vi "noindexString.vi"() -> ()   [LabVIEW 2020]
panel:
  out "number":u64[](array[numeric]) format="%.0x"
  out "Array":string[](array[string])
  in  "String":string
  out "Batch Length":i32
  out "Actual Bitrate kHz 2":i32=1000
  out "dup Cheetah Handle":i32
  out "Total Shifted Out":i32
  out "Actual Bitrate kHz":i32=1000
  out "error out":errorcluster
  in  "Rds per Sec":dbl=2000.0 max=2000000000.0
  out "SDO":u64[](array[numeric]) format="%x"
  in  "SCLK (kHz)":i32=2000 min=0
  out "Cheetah Handle":i32
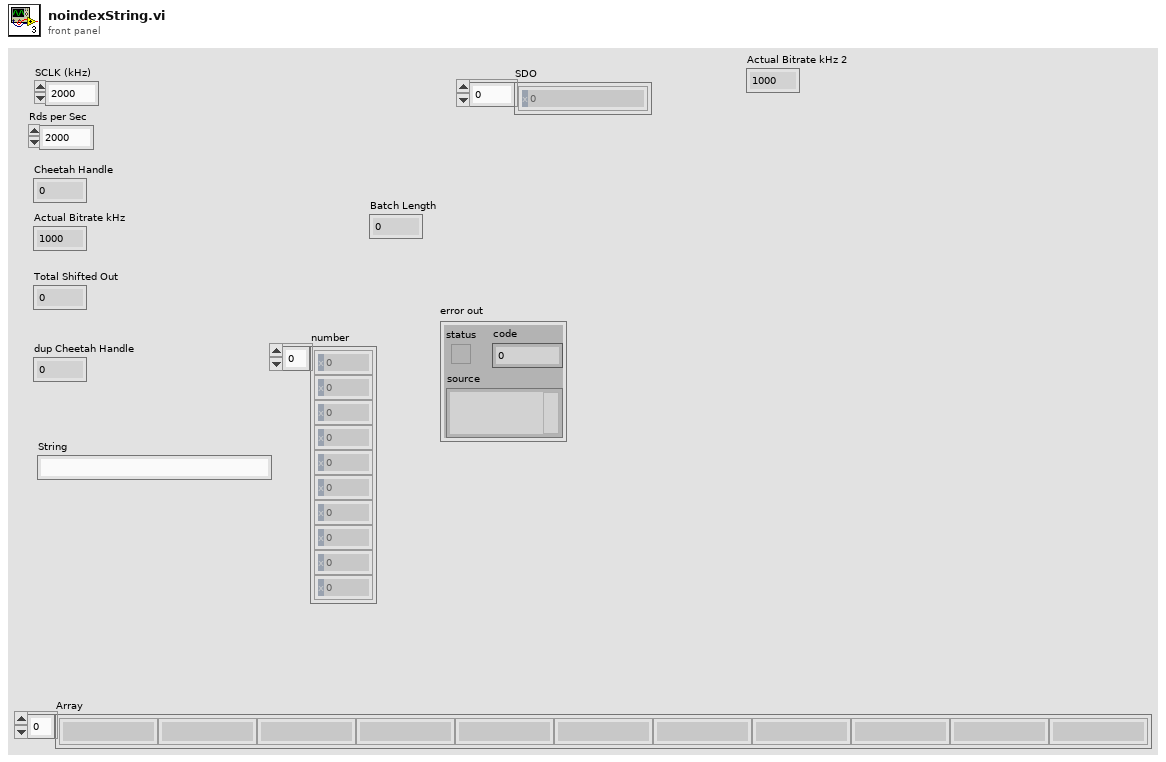
[diagram p1: front panel]
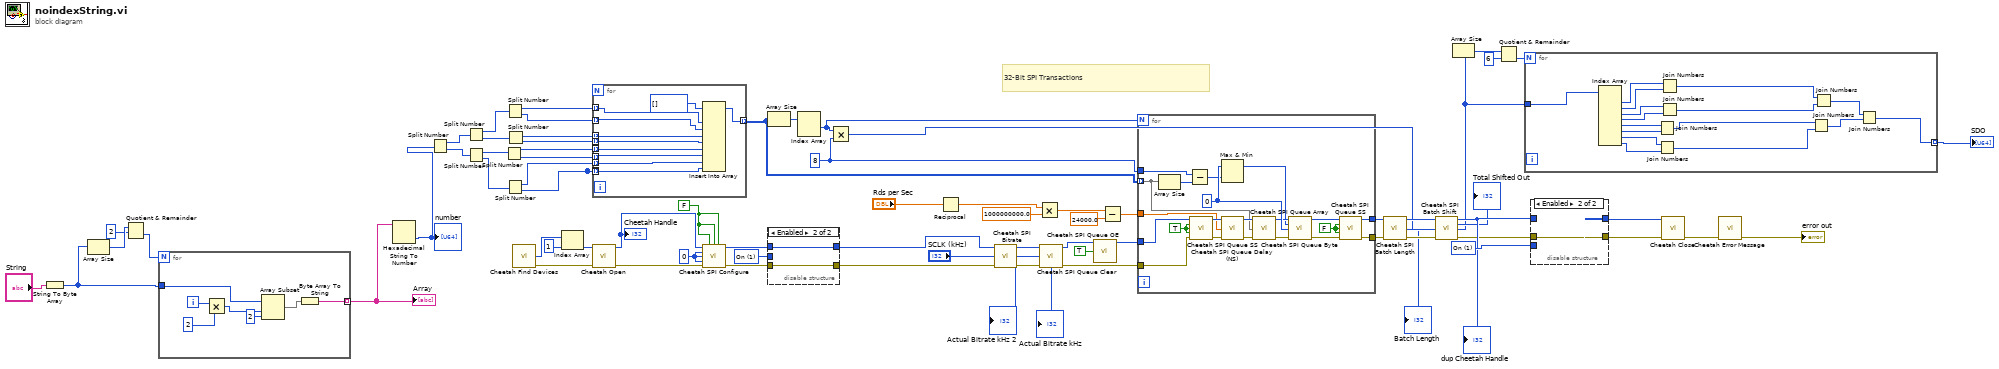
[diagram p0: block diagram]
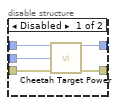
[diagram p2: hidden frame]
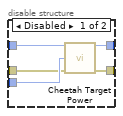
[diagram p3: hidden frame]
diagram:
  w26 = 8 ("y")
  w51 = u16 1 items=["Off", "On", "Query"] ("Requested Configuration (2: Query)")
  w52 = u16 1 items=["Off", "On", "Query"] ("Requested Configuration (2: Query)")
  w67 = FALSE
  w69 = 0
  # "32-Bit SPI Transactions"
  n1 = String To Byte Array(string="String") -> (unsigned byte array=w6:u8[])
  n2 = Array Size(array=w6) -> (size(s)=w5:i32)
  n3 = Quotient & Remainder(x=w5, y=2) -> (floor(x/y)=w3:i32)  [unwired: 1 out]
  n4 = for {
    N: w3 -> [_]
    tunnel: w6 -> [w78]
    tunnel: [w73] -> w2 mode=indexing
    i -> [w77]
    n5 = Multiply(x=w77, y=2) -> (x*y=w75:i32)
    n6 = Array Subset(array=w78, index=w75, length=2) -> (w72:u8[])
    n7 = Byte Array To String(unsigned byte array=w72) -> (string=w73:string)
  }
  "Array" <- w2
  n8 = Hexadecimal String To Number(string=w2) -> (number=w1:u32[])  [unwired: 2 in, 1 out]
  "number" <- w1
  n9 = Split Number(x=w1) -> (hi(x)=w37:u16[], lo(x)=w36:u16[])
  n10 = Split Number(x=w37) -> (hi(x)=w14:u8[], lo(x)=w13:u8[])
  n11 = Split Number(x=w36) -> (hi(x)=w16:u8[], lo(x)=w15:u8[])
  n12 = Split Number(x=w16) -> (hi(x)=w20:u8[], lo(x)=w19:u8[])
  n13 = Split Number(x=w14) -> (hi(x)=w12:u8[], lo(x)=w11:u8[])
  n14 = Split Number(x=w15) -> (hi(x)=w18:u8[], lo(x)=w17:u8[])
  n15 = Split Number(x=w13) -> (hi(x)=w10:u8[], lo(x)=w9:u8[])
  n16 = call <instrlib>:"Cheetah Find Devices.vi"() -> ("Ports"=w70:u16[], "error out"=w66:errorcluster)  [unwired: 13 in, 1 out]
  n17 = Index Array(array=w70, index=1) -> (element=w58:u16)
  n18 = for {
    tunnel: w20 -> [w88] mode=indexing
    tunnel: [w87] -> w35 mode=indexing
    tunnel: w18 -> [w85] mode=indexing
    tunnel: w17 -> [_] mode=indexing
    tunnel: w17 -> [w84] mode=indexing
    tunnel: w19 -> [w83] mode=indexing
    tunnel: w12 -> [w82] mode=indexing
    tunnel: w11 -> [w81] mode=indexing
    tunnel: w10 -> [w80] mode=indexing
    tunnel: w9 -> [w79] mode=indexing
    n19 = Insert Into Array(array=u8[] [], new element #1=w82, new element #2=w81, new element #3=w80, new element #4=w79, new element #5=w88, new element #6=w83, new element #7=w85, new element #8=w84) -> (w87:u8[])  [unwired: 1 in]
  }
  n20 = call <instrlib>:"Cheetah Open.vi"("Port Number (0)"=w58, "error in (no error)"=w66) -> ("Cheetah Handle"=w63:i32, "error out"=w65:errorcluster)  [unwired: 12 in]
  "Cheetah Handle" <- w63
  n21 = call <instrlib>:"Cheetah SPI Configure.vi"("Cheetah Handle"=w63, "SS0 Active High? (False)"=w67, "SS1 Active High? (False)"=w67, "SS2 Active High? (False)"=w67, "Polarity (0: Rising/Falling)"=w69, "Phase (0: Sample/Setup)"=w69, "Bitorder (0: MSB)"=w69, "error in (no error)"=w65) -> ("dup Cheetah Handle"=w62:i32, "error out"=w64:errorcluster)  [unwired: 6 in]
  n22 = disable-structure shown="Enabled" {
    disable-tunnel: w64 -> [w93 w94]
    disable-tunnel: w62 -> [w92 w95]
    disable-tunnel: [w91 w94] -> w61
    disable-tunnel: [w90 w95] -> w59
    disable-tunnel: w51 -> [w89 _]
    frame Disabled {
      n23 = call <instrlib>:"Cheetah Target Power.vi"("Cheetah Handle"=w92, "Requested Configuration (2: Query)"=w89, "error in (no error)"=w93) -> ("dup Cheetah Handle"=w90:i32, "error out"=w91:errorcluster)  [unwired: 10 in, 1 out]
    }
    frame Enabled {
    }
  }
  n24 = Array Size(array=w35) -> (size(s)=w50:i32[])
  n25 = Index Array(array=w50) -> (element #1=w22:i32)  [unwired: 2 in, 1 out]
  n26 = Multiply(x=w22, y=w26) -> (x*y=w21:i32)
  n27 = Reciprocal(x="Rds per Sec") -> (1/x=w28:dbl)
  n28 = call <instrlib>:"Cheetah SPI Bitrate.vi"("Cheetah Handle"=w59, "Requested Bitrate kHz (1000)"="SCLK (kHz)", "error in (no error)"=w61) -> ("dup Cheetah Handle"=w57:i32, "Actual Bitrate kHz"=→"Actual Bitrate kHz" →"Actual Bitrate kHz 2":i32, "error out"=w56:errorcluster)  [unwired: 10 in]
  n29 = Multiply(x=w28, y=1000000000.0) -> (x*y=w31:dbl)
  n30 = call <instrlib>:"Cheetah SPI Queue Clear.vi"("Cheetah Handle"=w57, "error in (no error)"=w56) -> ("dup Cheetah Handle"=w49:i32, "error out"=w68:errorcluster)  [unwired: 12 in]
  n31 = call <instrlib>:"Cheetah SPI Queue OE.vi"("Cheetah Handle"=w49, "Output Enable (on)"=TRUE) -> ("dup Cheetah Handle"=w48:i32)  [unwired: 12 in, 1 out]
  n32 = Subtract(x=w31, y=24000.0) -> (x-y=w29:dbl)
  n33 = for {
    N: w22 -> [_]
    tunnel: w68 -> [w102]
    tunnel: w48 -> [w103]
    tunnel: w35 -> [w104] mode=indexing
    tunnel: [w101] -> w46
    tunnel: [w100] -> w45
    tunnel: w29 -> [w97]
    tunnel: w26 -> [w98]
    w108 = FALSE
    w111 = 0
    w99 = TRUE
    n34 = Array Size(array=w104) -> (size(s)=w105:i32)
    n35 = Subtract(x=w98, y=w105) -> (x-y=w109:i32)
    n36 = call <instrlib>:"Cheetah SPI Queue SS.vi"("Cheetah Handle"=w103, "SS0 Assert? (True)"=w99, "SS1 Assert? (True)"=w99, "SS2 Assert? (True)"=w99, "error in (no error)"=w102) -> ("dup Cheetah Handle"=w116:i32, "error out"=w115:errorcluster)  [unwired: 9 in]
    n37 = Max & Min(x=w111, y=w109) -> (max(x,y)=w96:i32)  [unwired: 1 out]
    n38 = call <instrlib>:"Cheetah SPI Queue Delay (NS).vi"("Cheetah Handle"=w116, "Delay NS (1000)"=w97, "error in (no error)"=w115) -> ("dup Cheetah Handle"=w114:i32, "error out"=w113:errorcluster)  [unwired: 10 in, 1 out]
    n39 = call <instrlib>:"Cheetah SPI Queue Array.vi"("Cheetah Handle"=w114, "Data Out (none)"=w104, "error in (no error)"=w113) -> ("dup Cheetah Handle"=w110:i32, "error out"=w112:errorcluster)  [unwired: 11 in]
    n40 = call <instrlib>:"Cheetah SPI Queue Byte.vi"("Cheetah Handle"=w110, "Byte Count (1)"=w96, "Byte Value (0x00)"=w111, "error in (no error)"=w112) -> ("dup Cheetah Handle"=w107:i32, "error out"=w106:errorcluster)  [unwired: 10 in]
    n41 = call <instrlib>:"Cheetah SPI Queue SS.vi"("Cheetah Handle"=w107, "SS0 Assert? (True)"=w108, "SS1 Assert? (True)"=w108, "SS2 Assert? (True)"=w108, "error in (no error)"=w106) -> ("dup Cheetah Handle"=w100:i32, "error out"=w101:errorcluster)  [unwired: 9 in]
  }
  n42 = call <instrlib>:"Cheetah SPI Batch Length.vi"("Cheetah Handle"=w45, "error in (no error)"=w46) -> ("dup Cheetah Handle"=w44:i32, "Batch Length"=→"Batch Length":i32, "error out"=w43:errorcluster)  [unwired: 11 in]
  n43 = call <instrlib>:"Cheetah SPI Batch Shift.vi"("Cheetah Handle"=w44, "Max Bytes to Retrieve (256)"=w21, "error in (no error)"=w43) -> ("dup Cheetah Handle"=w42:i32, "Total Shifted Out"=→"Total Shifted Out":i32, "Data In"=w23:u8[], "error out"=w34:errorcluster)  [unwired: 9 in]
  "dup Cheetah Handle" <- w42
  n44 = Array Size(array=w23) -> (size(s)=w41:i32)
  n45 = Quotient & Remainder(x=w41, y=6) -> (floor(x/y)=w39:i32)  [unwired: 1 out]
  n46 = for {
    N: w39 -> [_]
    tunnel: w23 -> [w131]
    tunnel: [w130] -> w38 mode=indexing
    n47 = Index Array(array=w131) -> (element #1=w120:u8, element #2=w119:u8, element #3=w118:u8, element #4=w117:u8, element #5=w129:u8, element #6=w128:u8, element #7=w127:u8, element #8=w126:u8)  [unwired: 8 in]
    n48 = Join Numbers(hi=w129, lo=w128) -> ((hi.lo)=w125:u16)
    n49 = Join Numbers(hi=w127, lo=w126) -> ((hi.lo)=w124:u16)
    n50 = Join Numbers(hi=w120, lo=w119) -> ((hi.lo)=w123:u16)
    n51 = Join Numbers(hi=w118, lo=w117) -> ((hi.lo)=w122:u16)
    n52 = Join Numbers(hi=w125, lo=w124) -> ((hi.lo)=w132:u32)
    n53 = Join Numbers(hi=w123, lo=w122) -> ((hi.lo)=w121:u32)
    n54 = Join Numbers(hi=w121, lo=w132) -> ((hi.lo)=w130:u64)
  }
  "SDO" <- w38
  n55 = disable-structure shown="Enabled" {
    disable-tunnel: [w137 _] -> w55
    disable-tunnel: [w136 w138] -> w54
    disable-tunnel: w52 -> [w135 _]
    disable-tunnel: w42 -> [w134 _]
    disable-tunnel: w34 -> [w133 w138]
    frame Disabled {
      n56 = call <instrlib>:"Cheetah Target Power.vi"("Cheetah Handle"=w134, "Requested Configuration (2: Query)"=w135, "error in (no error)"=w133) -> ("dup Cheetah Handle"=w137:i32, "error out"=w136:errorcluster)  [unwired: 10 in, 1 out]
    }
    frame Enabled {
    }
  }
  n57 = call <instrlib>:"Cheetah Close.vi"("Cheetah Handle"=w55, "error in (no error)"=w54) -> ("error out"=w53:errorcluster)  [unwired: 12 in, 1 out]
  n58 = call <instrlib>:"Cheetah Error Message.vi"("error in (no error)"=w53) -> ("error out"=→"error out":errorcluster)  [unwired: 10 in, 4 out]
